vi "FT10_Log Update Mono1 Coag Log.vi"(10 "Mono1 Coag Activate":T1, 11 "Message Handling Cluster in":T2={"Fornax Connected?"=refnum, "Unitherm Connected?"=refnum, "M4X Connected?"=refnum, "Unitherm Connect/Disconnect"=refnum, "Fornax Connection"=refnum, "UNITHERM Connection"="", "M4X Connection"=0, "FPGA VI Reference Out"=refnum, "PXI-7854R Connected?"=refnum, "Fornax Connect/Disconnect"=refnum, "7854 Connect/Disconnect"=refnum, "M4X Connect/Disconnect"=refnum, "Config cluster"={"Unitherm Port"="", "Simulate Values"=FALSE, "Fornax Connect Attempts"=0}, "Log Queue"=refnum, "Log Analysis Cluster - Current"={"RMS"=0.0, "Envelope Frequency"=0.0, "Peak"=0.0, "Crest Factor"=0.0, "Duty Cyle %"=0.0, "P-P"=0.0, "Frequency"=0.0, "THD"=0.0, "Postive Peak"=0.0, "Negative Peak"=0.0, "Mag_H1"=0.0, "Phase_H1"=0.0, "Mag_H3"=0.0, "Phase_H3"=0.0, "Mag_H5"=0.0, "Phase_H5"=0.0}, "Log Waveform Cluster - Current"={"t0"=timestamp(0 s since 1904-01-01), "dt"=1.0, "Y"=[]}, "Log Time"=timestamp(0 s since 1904-01-01), "Log Flag"=FALSE, "Log - Activation Settings Cluster"={"Log - Unitherm Load"="", "Log - Port"="", "Log - Mode"="", "Log - Power Level"=""}, "Log - Port Mode Cluster"={"Mono1 Cut Enum"=enum."Pure", "Mono2 Cut Enum"=enum."Pure", "Mono1 Coag Enum"=enum."Fulgerate", "Mono2 Coag Enum"=enum."Fulgerate", "Bipolar Enum"=enum."Standard"}, "Log Analysis Cluster - Diff Voltage"={"RMS"=0.0, "Envelope Frequency"=0.0, "Peak"=0.0, "Crest Factor"=0.0, "Duty Cyle %"=0.0, "P-P"=0.0, "Frequency"=0.0, "THD"=0.0, "Postive Peak"=0.0, "Negative Peak"=0.0, "Mag_H1"=0.0, "Phase_H1"=0.0, "Mag_H3"=0.0, "Phase_H3"=0.0, "Mag_H5"=0.0, "Phase_H5"=0.0}, "Log Waveform Cluster - Diff Voltage"={"t0"=timestamp(0 s since 1904-01-01), "dt"=1.0, "Y"=[]}, "Indicator Cluster"={"Mono1 - Cut Power"=refnum, "Mono1 - Coag Power"=refnum, "Mono2 - Cut Power"=refnum, "Mono2 - Coag Power"=refnum, "Bipolar Power"=refnum, "Mono1 Cut Enum"=refnum, "Mono1 Coag Enum"=refnum, "Mono2 Cut Enum"=refnum, "Mono2 Coag Enum"=refnum, "Bipolar Enum"=refnum}, "Log Power Level Cluster"={"Log Mono1 Cut Power"="", "Log Mono1 Coag Power"="", "Log Mono2 Cut Power"="", "Log Mono2 Coag Power"="", "Log Bipolar Power"=""}, "Footswitch Cluster"={"PXI-2565 reset device (boolean value)"=TRUE, "topology name"="2565/16-SPST", "PXI-2565 simulate (boolean value)"=FALSE, "PXI-2565 resource name"=""}}) -> (3 "Message Handling Cluster out":T2={"Fornax Connected?"=refnum, "Unitherm Connected?"=refnum, "M4X Connected?"=refnum, "Unitherm Connect/Disconnect"=refnum, "Fornax Connection"=refnum, "UNITHERM Connection"="", "M4X Connection"=0, "FPGA VI Reference Out"=refnum, "PXI-7854R Connected?"=refnum, "Fornax Connect/Disconnect"=refnum, "7854 Connect/Disconnect"=refnum, "M4X Connect/Disconnect"=refnum, "Config cluster"={"Unitherm Port"="", "Simulate Values"=FALSE, "Fornax Connect Attempts"=0}, "Log Queue"=refnum, "Log Analysis Cluster - Current"={"RMS"=0.0, "Envelope Frequency"=0.0, "Peak"=0.0, "Crest Factor"=0.0, "Duty Cyle %"=0.0, "P-P"=0.0, "Frequency"=0.0, "THD"=0.0, "Postive Peak"=0.0, "Negative Peak"=0.0, "Mag_H1"=0.0, "Phase_H1"=0.0, "Mag_H3"=0.0, "Phase_H3"=0.0, "Mag_H5"=0.0, "Phase_H5"=0.0}, "Log Waveform Cluster - Current"={"t0"=timestamp(0 s since 1904-01-01), "dt"=1.0, "Y"=[]}, "Log Time"=timestamp(0 s since 1904-01-01), "Log Flag"=FALSE, "Log - Activation Settings Cluster"={"Log - Unitherm Load"="", "Log - Port"="", "Log - Mode"="", "Log - Power Level"=""}, "Log - Port Mode Cluster"={"Mono1 Cut Enum"=enum."Pure", "Mono2 Cut Enum"=enum."Pure", "Mono1 Coag Enum"=enum."Fulgerate", "Mono2 Coag Enum"=enum."Fulgerate", "Bipolar Enum"=enum."Standard"}, "Log Analysis Cluster - Diff Voltage"={"RMS"=0.0, "Envelope Frequency"=0.0, "Peak"=0.0, "Crest Factor"=0.0, "Duty Cyle %"=0.0, "P-P"=0.0, "Frequency"=0.0, "THD"=0.0, "Postive Peak"=0.0, "Negative Peak"=0.0, "Mag_H1"=0.0, "Phase_H1"=0.0, "Mag_H3"=0.0, "Phase_H3"=0.0, "Mag_H5"=0.0, "Phase_H5"=0.0}, "Log Waveform Cluster - Diff Voltage"={"t0"=timestamp(0 s since 1904-01-01), "dt"=1.0, "Y"=[]}, "Indicator Cluster"={"Mono1 - Cut Power"=refnum, "Mono1 - Coag Power"=refnum, "Mono2 - Cut Power"=refnum, "Mono2 - Coag Power"=refnum, "Bipolar Power"=refnum, "Mono1 Cut Enum"=refnum, "Mono1 Coag Enum"=refnum, "Mono2 Cut Enum"=refnum, "Mono2 Coag Enum"=refnum, "Bipolar Enum"=refnum}, "Log Power Level Cluster"={"Log Mono1 Cut Power"="", "Log Mono1 Coag Power"="", "Log Mono2 Cut Power"="", "Log Mono2 Coag Power"="", "Log Bipolar Power"=""}, "Footswitch Cluster"={"PXI-2565 reset device (boolean value)"=TRUE, "topology name"="2565/16-SPST", "PXI-2565 simulate (boolean value)"=FALSE, "PXI-2565 resource name"=""}})   [LabVIEW 2024]
doc: "Update \"Log Activation Settings Cluster\" with the Mono1 - Coag Port and its Mode."
uses:
  Controls/Control_Message Handling Cluster.ctl
  Controls/Control_M4X Connection.ctl
  Controls/Control_PXI-7854R FPGA Reference.ctl
  Controls/Control_Config Cluster.ctl
  Controls/Control_Config Unitherm Port.ctl
  Controls/Control_Config Simulate Values.ctl
  Controls/Control_Config Fornax Connect Attempts.ctl
  Controls/Control_Log Queue.ctl
  Controls/Control_Log Cluster.ctl
  Controls/Control_Log Time.ctl
  Controls/Control_Log Waveform Cluster - Current.ctl
  Controls/Control_Log Analysis Cluster - Current.ctl
  Controls/Control_Log Activation Settings Cluster.ctl
  Controls/Control_Log Unitherm Load.ctl
  Controls/Control_Log Port.ctl
  Controls/Control_Log Mode.ctl
  Controls/Control_Log Power Level.ctl
  Controls/Control_Log Waveform Cluster - Diff Voltage.ctl
  Controls/Control_Log Analysis Cluster - Diff Voltage.ctl
  Controls/Control_Log Flag.ctl
  Controls/Control_Log Port Mode Cluster.ctl
  Controls/Control_Fornax Mono1 Cut Enum.ctl
  Controls/Control_Fornax Mono2 Cut Enum.ctl
  Controls/Control_Fornax Mono1 Coag Enum.ctl
  Controls/Control_Fornax Mono2 Coag Enum.ctl
  Controls/Control_Fornax Bipolar Enum.ctl
  Controls/Control_Indicator Cluster.ctl
  Controls/Control_Log Power Level Cluster.ctl
  Controls/Control_Log Mono1 Cut Power.ctl
  Controls/Control_Log Mono1 Coag Power.ctl
  Controls/Control_Log Mono2 Cut Power.ctl
  Controls/Control_Log Mono2 Coag Power.ctl
  Controls/Control_Log Bipolar Power.ctl
  Controls/Control_Footswitch Reset Device Bool.ctl
  <instrlib>/niSwitch/niSwitch.llb/niSwitch Topologies.ctl
  Controls/Control_Footswitch Simulate Bool.ctl
  Controls/Control_Footswitch Resource Name.ctl
  Controls/Control_Fornax Mono1 Coag Activate Port Bool.ctl
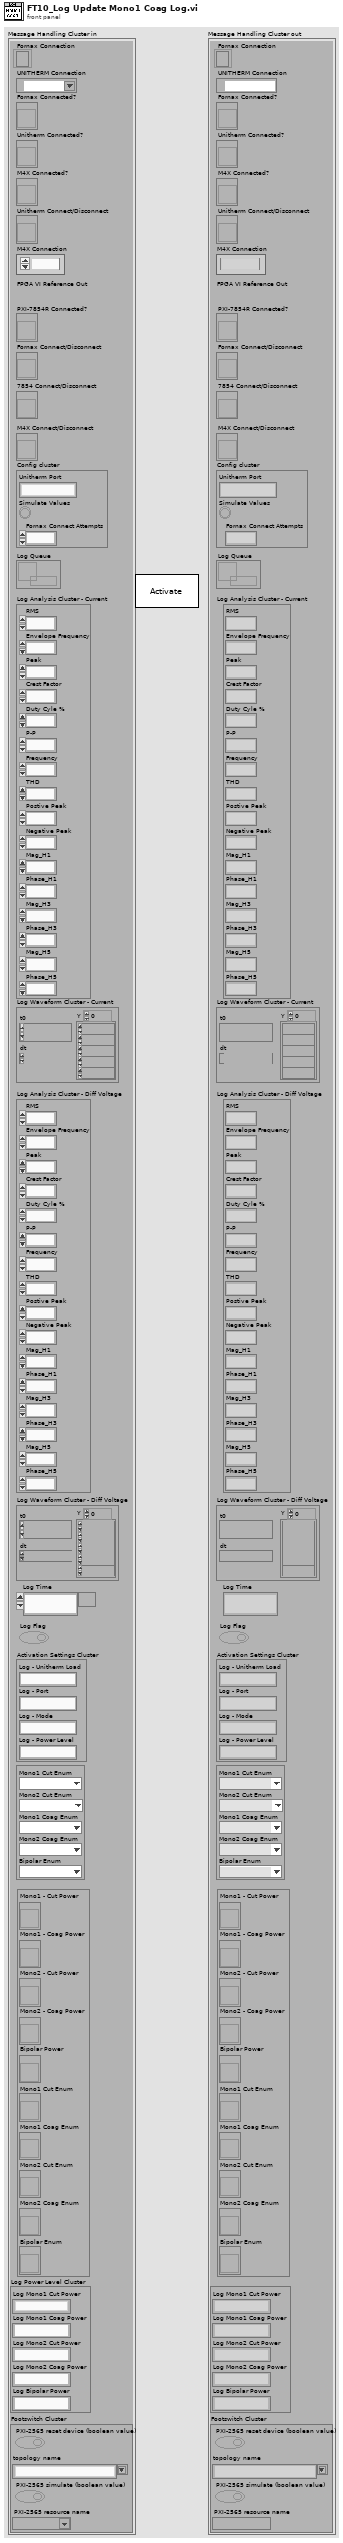
[diagram p1: front panel]
types:
  T1 = typedef "Control_Fornax Mono1 Coag Activate Port Bool.ctl" = bool
  T2 = typedef "Control_Message Handling Cluster.ctl" = cluster{"Fornax Connected?":refnum<vi>, "Unitherm Connected?":refnum<vi>, "M4X Connected?":refnum<vi>, "Unitherm Connect/Disconnect":refnum<vi>, "Fornax Connection":refnum<k5>, "UNITHERM Connection":refnum<visa-resource-name>, "M4X Connection":T3, "FPGA VI Reference Out":T4, "PXI-7854R Connected?":refnum<vi>, "Fornax Connect/Disconnect":refnum<vi>, "7854 Connect/Disconnect":refnum<vi>, "M4X Connect/Disconnect":refnum<vi>, "Config cluster":T5, "Log Queue":T9, "Log Analysis Cluster - Current":T10, "Log Waveform Cluster - Current":T11, "Log Time":T12, "Log Flag":T13, "Log - Activation Settings Cluster":T14, "Log - Port Mode Cluster":T19, "Log Analysis Cluster - Diff Voltage":T25, "Log Waveform Cluster - Diff Voltage":T26, "Indicator Cluster":T27, "Log Power Level Cluster":T28, "Footswitch Cluster":cluster{"PXI-2565 reset device (boolean value)":T34, "topology name":T35, "PXI-2565 simulate (boolean value)":T36, "PXI-2565 resource name":T37}}
  T3 = typedef "Control_M4X Connection.ctl" = u32
  T4 = typedef "Control_PXI-7854R FPGA Reference.ctl" = refnum<k20>
  T5 = typedef "Control_Config Cluster.ctl" = cluster{"Unitherm Port":T6, "Simulate Values":T7, "Fornax Connect Attempts":T8}
  T6 = typedef "Control_Config Unitherm Port.ctl" = string
  T7 = typedef "Control_Config Simulate Values.ctl" = bool
  T8 = typedef "Control_Config Fornax Connect Attempts.ctl" = i32
  T9 = typedef "Control_Log Queue.ctl" = refnum<queue>
  T10 = typedef "Control_Log Analysis Cluster - Current.ctl" = cluster{"RMS":dbl, "Envelope Frequency":dbl, "Peak":dbl, "Crest Factor":dbl, "Duty Cyle %":dbl, "P-P":dbl, "Frequency":dbl, "THD":dbl, "Postive Peak":dbl, "Negative Peak":dbl, "Mag_H1":dbl, "Phase_H1":dbl, "Mag_H3":dbl, "Phase_H3":dbl, "Mag_H5":dbl, "Phase_H5":dbl}
  T11 = typedef "Control_Log Waveform Cluster - Current.ctl" = waveform(dbl)
  T12 = typedef "Control_Log Time.ctl" = timestamp
  T13 = typedef "Control_Log Flag.ctl" = bool
  T14 = typedef "Control_Log Activation Settings Cluster.ctl" = cluster{"Log - Unitherm Load":T15, "Log - Port":T16, "Log - Mode":T17, "Log - Power Level":T18}
  T15 = typedef "Control_Log Unitherm Load.ctl" = string
  T16 = typedef "Control_Log Port.ctl" = string
  T17 = typedef "Control_Log Mode.ctl" = string
  T18 = typedef "Control_Log Power Level.ctl" = string
  T19 = typedef "Control_Log Port Mode Cluster.ctl" = cluster{"Mono1 Cut Enum":T20, "Mono2 Cut Enum":T21, "Mono1 Coag Enum":T22, "Mono2 Coag Enum":T23, "Bipolar Enum":T24}
  T20 = typedef "Control_Fornax Mono1 Cut Enum.ctl" = enum16{"Pure", "Blend"}
  T21 = typedef "Control_Fornax Mono2 Cut Enum.ctl" = enum16{"Pure", "Blend"}
  T22 = typedef "Control_Fornax Mono1 Coag Enum.ctl" = enum16{"Fulgerate", "Spray"}
  T23 = typedef "Control_Fornax Mono2 Coag Enum.ctl" = enum16{"Fulgerate", "Spray"}
  T24 = typedef "Control_Fornax Bipolar Enum.ctl" = enum16{"Standard", "Macro", "Precision"}
  T25 = typedef "Control_Log Analysis Cluster - Diff Voltage.ctl" = cluster{"RMS":dbl, "Envelope Frequency":dbl, "Peak":dbl, "Crest Factor":dbl, "Duty Cyle %":dbl, "P-P":dbl, "Frequency":dbl, "THD":dbl, "Postive Peak":dbl, "Negative Peak":dbl, "Mag_H1":dbl, "Phase_H1":dbl, "Mag_H3":dbl, "Phase_H3":dbl, "Mag_H5":dbl, "Phase_H5":dbl}
  T26 = typedef "Control_Log Waveform Cluster - Diff Voltage.ctl" = waveform(dbl)
  T27 = typedef "Control_Indicator Cluster.ctl" = cluster{"Mono1 - Cut Power":refnum<vi>, "Mono1 - Coag Power":refnum<vi>, "Mono2 - Cut Power":refnum<vi>, "Mono2 - Coag Power":refnum<vi>, "Bipolar Power":refnum<vi>, "Mono1 Cut Enum":refnum<vi>, "Mono1 Coag Enum":refnum<vi>, "Mono2 Cut Enum":refnum<vi>, "Mono2 Coag Enum":refnum<vi>, "Bipolar Enum":refnum<vi>}
  T28 = typedef "Control_Log Power Level Cluster.ctl" = cluster{"Log Mono1 Cut Power":T29, "Log Mono1 Coag Power":T30, "Log Mono2 Cut Power":T31, "Log Mono2 Coag Power":T32, "Log Bipolar Power":T33}
  T29 = typedef "Control_Log Mono1 Cut Power.ctl" = string
  T30 = typedef "Control_Log Mono1 Coag Power.ctl" = string
  T31 = typedef "Control_Log Mono2 Cut Power.ctl" = string
  T32 = typedef "Control_Log Mono2 Coag Power.ctl" = string
  T33 = typedef "Control_Log Bipolar Power.ctl" = string
  T34 = typedef "Control_Footswitch Reset Device Bool.ctl" = bool
  T35 = typedef "niSwitch Topologies.ctl" = string
  T36 = typedef "Control_Footswitch Simulate Bool.ctl" = bool
  T37 = typedef "Control_Footswitch Resource Name.ctl" = refnum<k15>
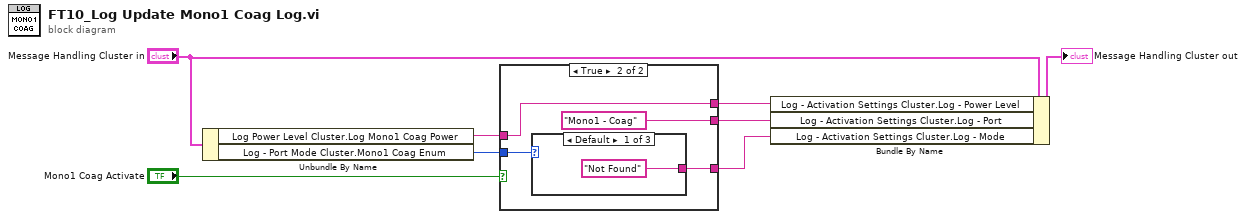
[diagram p0: block diagram]
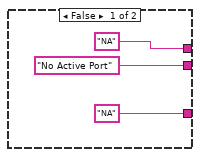
[diagram p2: hidden frame]
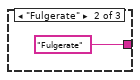
[diagram p3: hidden frame]
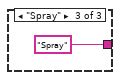
[diagram p4: hidden frame]
diagram:
  n1 = Unbundle By Name("Message Handling Cluster in") -> ("Log Power Level Cluster.Log Mono1 Coag Power"=w1:T30, "Log - Port Mode Cluster.Mono1 Coag Enum"=w5:T22)
  n2 = case shown="True" "Mono1 Coag Activate" {
    tunnel: w5 -> [_ w15]
    tunnel: [T16 "No Active Port" ("Log - Activation Settings Cluster.Log - Port") T16 "Mono1 - Coag" ("Log - Activation Settings Cluster.Log - Port")] -> w6
    tunnel: [T17 "NA" ("Log - Activation Settings Cluster.Log - Mode") w13] -> w7
    tunnel: [T18 "NA" ("Log - Activation Settings Cluster.Log - Power Level") w12] -> w2
    tunnel: w1 -> [_ w12]
    frame False {
    }
    frame True {
      n3 = case shown="Default" w15 {
        tunnel: [T17 "Not Found" ("Log - Activation Settings Cluster.Log - Mode") T17 "Fulgerate" ("Log - Activation Settings Cluster.Log - Mode") T17 "Spray" ("Log - Activation Settings Cluster.Log - Mode")] -> w13
        frame Default {
        }
        frame "Fulgerate" {
        }
        frame "Spray" {
        }
      }
    }
  }
  n4 = Bundle By Name(cluster="Message Handling Cluster in", "Log - Activation Settings Cluster.Log - Power Level"=w2, "Log - Activation Settings Cluster.Log - Port"=w6, "Log - Activation Settings Cluster.Log - Mode"=w7) -> (→"Message Handling Cluster out":T2)
